vi "Posiion rediction.vi"(9 "Current Position":T1) -> (0 "Hover Out":bool, 1 "Predicted Position":T1)   [LabVIEW 2014]
uses:
  Others/Global.vi
panel:
  out "Boolean":bool
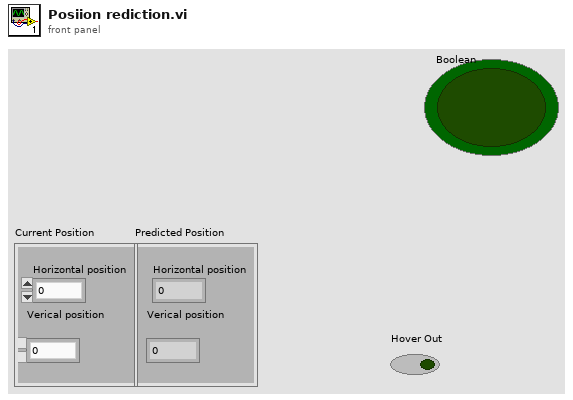
[diagram p1: front panel]
types:
  T1 = cluster{"Horizontal position":dbl, "Verical position\n":dbl}
  T2 = typedef "AR Drone.lvlib/NavData Demo.ctl" = cluster{"control state":enum32{"DEFAULT", "INIT", "LANDING", "FLYING", "HOVERING", "TEST", "TRANS_TAKEOFF", "TRANS_GOTOFIX", "TRANS_LANDING"}, "battery percentage":u32, "pitch (deg)":sgl, "roll (deg)":sgl, "yaw (deg)":sgl, "altitude (cm)":u32, "vx (cm/s)?":sgl, "vy (cm/s)?":sgl, "vz (cm/s)?":sgl, "detection cam type":u32}
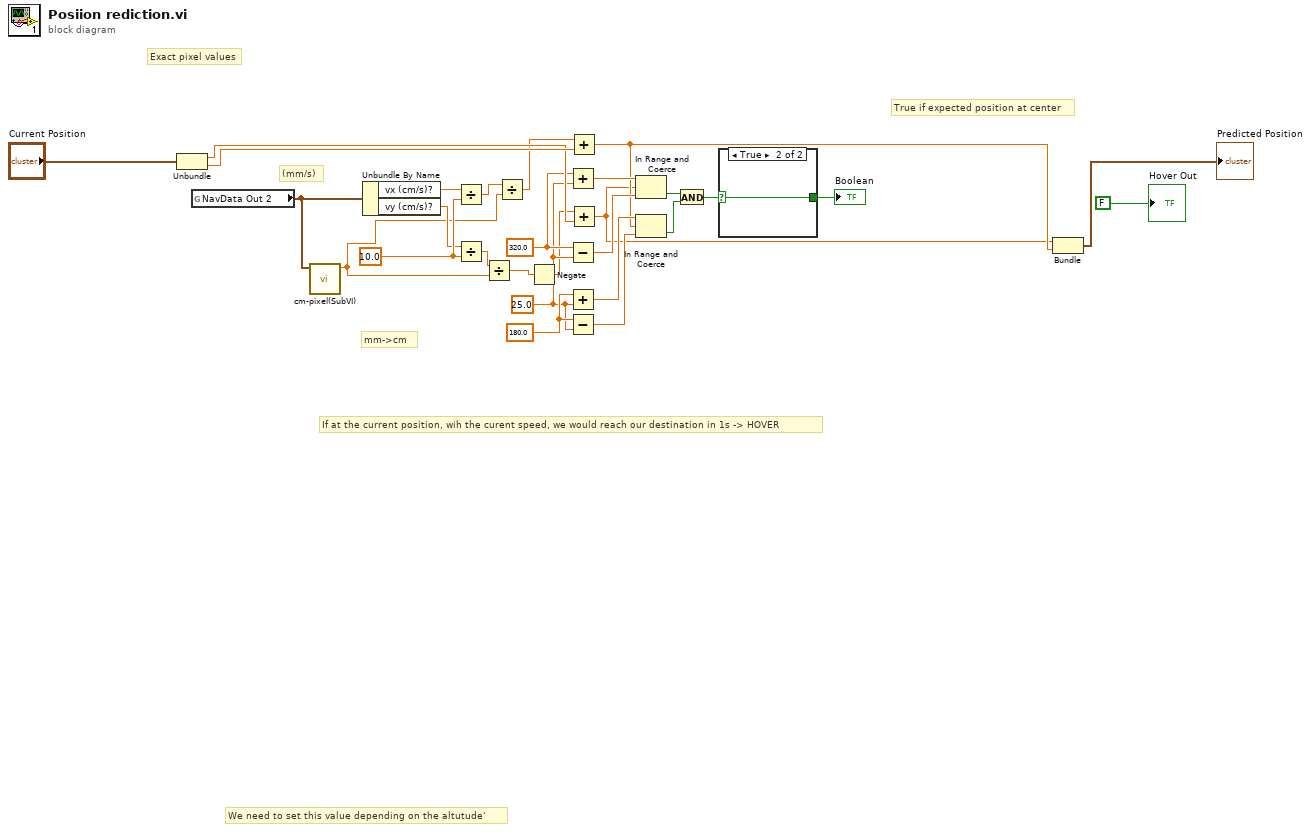
[diagram p0: block diagram]
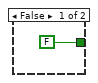
[diagram p2: hidden frame]
diagram:
  w20 = sgl 10.0 ("mm to cm")
  w12 = 180.0 ("upper limit")
  w13 = 320.0 ("upper limit")
  w11 = 25.0 ("upper limit")
  # "mm->cm"
  # "Exact pixel values"
  # "(mm/s)"
  # "True if expected position at center"
  # "We need to set this value depending on the altutude'"
  # "If at the current position, wih the curent speed, we would reach our destination in 1s -> HOVER"
  n1 = Unbundle("Current Position") -> ("Horizontal position"=w18:dbl, "Verical position"=w19:dbl)
  n2 = global read "Global.vi" "NavData Out 2"() -> (w21:T2)
  n3 = call "cm-pixel(SubVI).vi"("NavData Out in"=w21) -> ("1 pixel equals to: (in cm)"=w3:dbl)  [unwired: 10 in]
  n4 = Unbundle By Name(w21) -> ("vx (cm/s)?"=w8:sgl, "vy (cm/s)?"=w7:sgl)
  n5 = Divide(x=w8, y=w20) -> (x/y=w5:sgl)
  n6 = Divide(x=w7, y=w20) -> (x/y=w4:sgl)
  n7 = Divide(x=w4, y=w3) -> (x/y=w1:dbl)
  n8 = Divide(x=w5, y=w3) -> (x/y=w2:dbl)
  n9 = Negate(x=w1) -> (-x=w6:dbl)
  n10 = Add(x=w13, y=w11) -> (x+y=w14:dbl)
  n11 = Subtract(x=w13, y=w11) -> (x-y=w15:dbl)
  n12 = Add(x=w12, y=w11) -> (x+y=w16:dbl)
  n13 = Subtract(x=w12, y=w11) -> (x-y=w17:dbl)
  n14 = Add(x=w2, y=w19) -> (x+y=w10:dbl)
  n15 = Add(x=w6, y=w18) -> (x+y=w9:dbl)
  n16 = In Range and Coerce(upper limit=w14, x=w9, lower limit=w15) -> (In Range?=w23:bool)  [unwired: 1 out]
  n17 = In Range and Coerce(upper limit=w16, x=w10, lower limit=w17) -> (In Range?=w24:bool)  [unwired: 1 out]
  n18 = And(x=w23, y=w24) -> (x .and. y?=w25:bool)
  n19 = case shown="True" w25 {
    selector: w25 -> [_ w30]
    tunnel: [FALSE w30] -> w22
    frame False {
    }
    frame True {
    }
  }
  "Boolean" <- w22
  n20 = Bundle(w9, w10) -> (→"Predicted Position":cluster{dbl, dbl})  [unwired: 1 in]
  "Hover Out" <- FALSE ("Hover")
